vi "Freigabe Daten loggen.vi"() -> (1 "Daten loggen":bool)   [LabVIEW 2020, in "Messdaten.lvlib"]
uses:
  Messdaten.lvlib
  Funktionstasten/Funktionstasten-Aktion.ctl
  Funktionstasten/Zustaende.ctl
  Seiten/System Einstellungen V2/Aktioen FGV System.ctl
  Funktionstasten/Funktionstasten.lvlib
  Seiten/System Einstellungen V2/System Einstellungen V2.lvlib
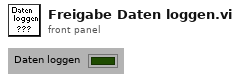
[diagram p1: front panel]
types:
  T1 = typedef "System Einstellungen V2.lvlib/Aktioen FGV System.ctl" = enum16{"lesen", "laden", "speichern", "Optionen schreiben", "Zeitstempel", "Reset BMP", "Reset SQP", "Wartung", "Werkseinstellung"}
  T2 = typedef "Funktionstasten.lvlib/Zustaende.ctl" = enum16{"Standby", "Pause", "Eco", "Messen", "Kalibrieren", "Spülen Filter", "Spülen Leitung", "Umgebungsluft", "0-Gas", "Cal-Gas", "CG zu PNS", "-------------", "Init 1", "Init 2", "Init 3", "Init 4", "Messen vorbereiten", "Messen durchführen", "Exit"}
  T3 = typedef "Funktionstasten.lvlib/Funktionstasten-Aktion.ctl" = enum16{"Initialisieren", "Zustand setzen", "Taste gedrückt", "Fehler speichern", "Lesen", "Manuell", "Remote", "Bitparallel", "Samplepoint", "Zeit Prüfen", "reset Umschalten"}
  T4 = typedef "System Einstellungen V2.lvlib/Optionen.ctl" = cluster{"Störmeldep.":bool, "Betriebszustände":bool, "AK in ppm":bool, "log Cal-Gas":bool, "log 0-Gas":bool, "Durchflusssensor 0-5V":bool, "PNS?":bool, "Mit N2 spülen":bool, "TRE08":bool, "Amium 10-Fach":bool, "Verticale Scrollbar aktiv":bool, "Loggingtakt":bool, "AK Rezeptwechsel gleich wie MKS":bool, "NG ECO":bool}
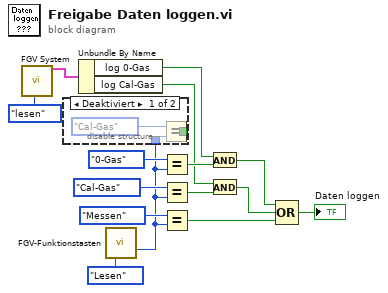
[diagram p0: block diagram]
diagram:
  n1 = call "FGV System.vi"("Aktionen"=Aktioen_FGV_System."lesen") -> ("Optionen"=w10:T4)  [unwired: 12 in, 6 out]
  n2 = Unbundle By Name(w10) -> ("log 0-Gas"=w6:bool, "log Cal-Gas"=w7:bool)
  n3 = call "FGV-Funktionstasten.vi"("Aktion"=Funktionstasten-Aktion."Lesen") -> ("ausgewählte Funktion"=w1:T2)  [unwired: 7 in, 7 out]
  n4 = disable-structure shown="Deaktiviert" {
    disable-tunnel: w1 -> [w17 _]
    disable-tunnel: [w16 _] -> _
    frame Disabled {
      n5 = Equal?(x=Zustaende."Cal-Gas" ("Zustand"), y=w17) -> (x = y?=w16:bool)
    }
    frame Enabled {
    }
  }
  n6 = Equal?(x=Zustaende."0-Gas" ("Zustand"), y=w1) -> (x = y?=w9:bool)
  n7 = Equal?(x=Zustaende."Cal-Gas" ("Zustand"), y=w1) -> (x = y?=w8:bool)
  n8 = Equal?(x=Zustaende."Messen" ("Zustand"), y=w1) -> (x = y?=w14:bool)
  n9 = And(x=w6, y=w9) -> (x .and. y?=w4:bool)
  n10 = And(x=w7, y=w8) -> (x .and. y?=w5:bool)
  n11 = Compound Arithmetic op=OR(w4, w5, w14) -> (→"Daten loggen":bool)
